vi "DSDLL Signalize Abort to Digitizing Process.vi"(8 "error in":errorcluster, 10 "send abort signal? (True)":bool=TRUE, 11 "dsdll in":T1) -> (0 "error out (copy)":errorcluster, 3 "dsdll out (copy)":T1)   [LabVIEW 2020, in "DSDLL Virtual Digitizer.lvlib"]
doc: "This will signalize abort action to the digitizing process. When this is called continue fetching as ussual until fetch VI returnes 'fetching done?' flag. If some data were already digitized it will be returned. The VI ignroes input error and will not generate any error."
uses:
  DSDLL Virtual Digitizer.lvlib
  DSDLL Session.ctl
  dsdll/dsdll_instance.ctl
  dsdll/dsdll_device_record.ctl
  DSDLL Process Config.ctl
  DSDLL Data Packet.ctl
  dsdll/dsdll.lvlib
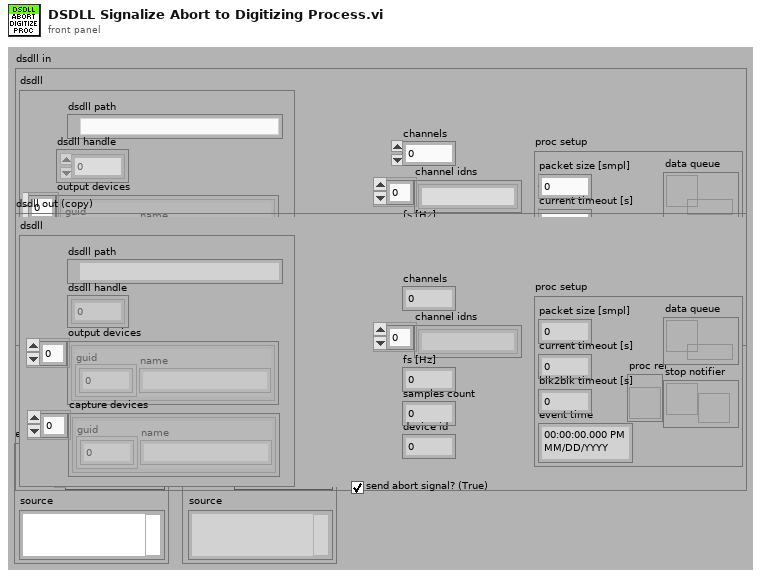
[diagram p1: front panel]
types:
  T1 = typedef "DSDLL Virtual Digitizer.lvlib/DSDLL Session.ctl" = cluster{"dsdll":T2, "channels":i32, "device id":i32, "channel idns":string[], "proc setup":T4, "samples count":i32, "fs [Hz]":dbl}
  T2 = typedef "dsdll.lvlib/dsdll_instance.ctl" = cluster{"dsdll path":path, "dsdll handle":u8[], "output devices":T3[], "capture devices":T3[]}
  T3 = typedef "dsdll.lvlib/dsdll_device_record.ctl" = cluster{"guid":u8[], "name":string}
  T4 = typedef "DSDLL Virtual Digitizer.lvlib/DSDLL Process Config.ctl" = cluster{"packet size [smpl]":i32, "current timeout [s]":dbl, "blk2blk timeout [s]":dbl, "event time":timestamp, "data queue":refnum<queue>, "stop notifier":refnum<notifier>, "proc ref":refnum<vi>}
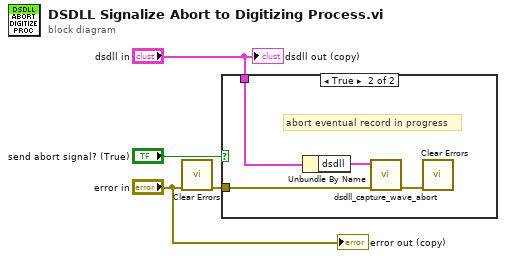
[diagram p0: block diagram]
diagram:
  n1 = call <vilib>:"Clear Errors.vi"("error in (no error)"="error in") -> ("error out"=w1:errorcluster)  [unwired: 5 in, 1 out]
  n2 = case shown="True" "send abort signal? (True)" {
    tunnel: w1 -> [_ w6]
    tunnel: "dsdll in" -> [_ w8]
    frame False {
    }
    frame True {
      # "abort eventual record in progress"
      n3 = Unbundle By Name(w8) -> ("dsdll"=w7:T2)
      n4 = call "dsdll_capture_wave_abort.vi"("error in"=w6, "dsdll instance in"=w7) -> ("error out"=w5:errorcluster)  [unwired: 7 in, 2 out]
      n5 = call <vilib>:"Clear Errors.vi"("error in (no error)"=w5) -> ()  [unwired: 5 in, 2 out]
    }
  }
  "error out (copy)" <- "error in"
  "dsdll out (copy)" <- "dsdll in"
